vi "ParBRecv.vi"(0 "ref in":u64, 9 "data in":string, 11 "error in (no error)":errorcluster) -> (4 "ref out":u64, 6 "Result":i32, 8 "DataReady":bool, 10 "data out":string, 12 "R_ID":u32, 13 "Size":i32, 15 "error out":errorcluster)   [LabVIEW 2019, in "Snap7.lvlib"]
uses:
  Snap7.lvlib
  windows/lv_snap7.dll
panel:
  in  "var DataReady":i32
  in  "var Size":i32
  in  "var R_ID":u32=1
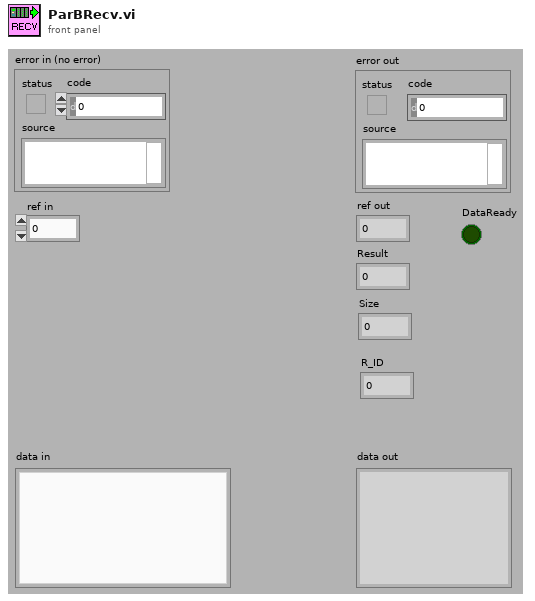
[diagram p1: front panel]
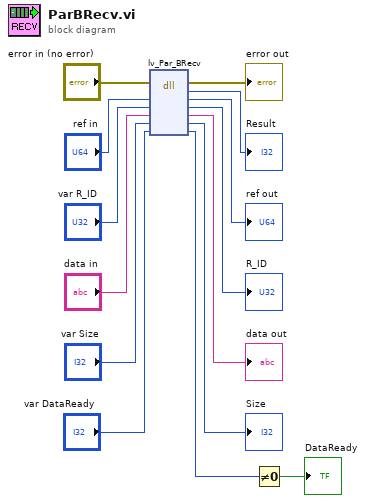
[diagram p0: block diagram]
diagram:
  n1 = dll-call lib="PTH2Xabs DSVNHLCEPStrunk性能试验台SourcesSnap7libwindowslv_snap7.dll" fn="lv_Par_BRecv"(error in="error in (no error)", "Partner"="ref in", "R_ID"="var R_ID", "pUsrData"="data in", "Size"="var Size", "DataReady"="var DataReady") -> (error out=→"error out":errorcluster, "return type"=→"Result":i32, "Partner"=→"ref out":u64, "R_ID"=→"R_ID":u32, "pUsrData"=→"data out":string, "Size"=→"Size":i32, "DataReady"=w2:i32)  [unwired: 2 in, 1 out]
  n2 = Not Equal To 0?(x=w2) -> (x != 0?=→"DataReady":bool)
